vi "AutoApproach.vi"() -> ()   [LabVIEW 2014]
uses:
  <vilib>/userdefined/High Color/nirio_resource_hc.ctl
  <vilib>/Instr/_visa.llb/VISA Configure Serial Port (Instr).vi
  <vilib>/FPGAPlugInAG/PCIe-7851R/niLvFpga_Open_PCIe-7851R.vi
  <vilib>/rvi/interface/common/dynamic/niFpgaDynamicAddResources.vi
  <vilib>/Utility/error.llb/Error Cluster From Error Code.vi
  <vilib>/rvi/errors/niLvFpgaAdjustHostInterfaceError.vi
  <vilib>/FPGAPlugInAG/Dynamic/niLvFpga_Close_Dynamic.vi
  <vilib>/rvi/interface/nirviOpenFPGA/nirviOpenFPGA.xnode
  FPGA Bitfiles/FastHoppingModel_FPGATarget_CurrRefFres_BupT8kKEpOg.lvbitx
  <vilib>/rvi/interface/nirviReadWriteControl/nirviReadWriteControl.xnode
  <vilib>/rvi/interface/nirviCloseFPGA/nirviCloseFPGA.xnode
  FPGA Bitfiles/FastHoppingModel_FPGATarget_SingleApproach_ZxUoy3UGE18.lvbitx
  NiFpgaLv.dll
  <vilib>/rvi/interface/Simulation/niFpgaSimulationCallBeginRW.vi
panel:
  in  "RoughZOffset um":dbl format="%#_13g"
  out "Approached?":bool
  out "ERROut?":string
  in  "stop":bool
  out "RealPosIndex":i16
  out "preCurrIndex":i16
  out "PIZPosIndex":i16
  out "CurrDia":i16(graph)
  out "PIZPosDia":i16(graph)
  in  "Decline %":sgl format="%#_13g"
  in  "AppRate us":i32
  in  "BaseTime us":i32
  in  "PIZ":T1
  out "RoughZPos":dbl
  out "ERRIn?":string
  in  "RoughXYZ":refnum<visa-resource-name>
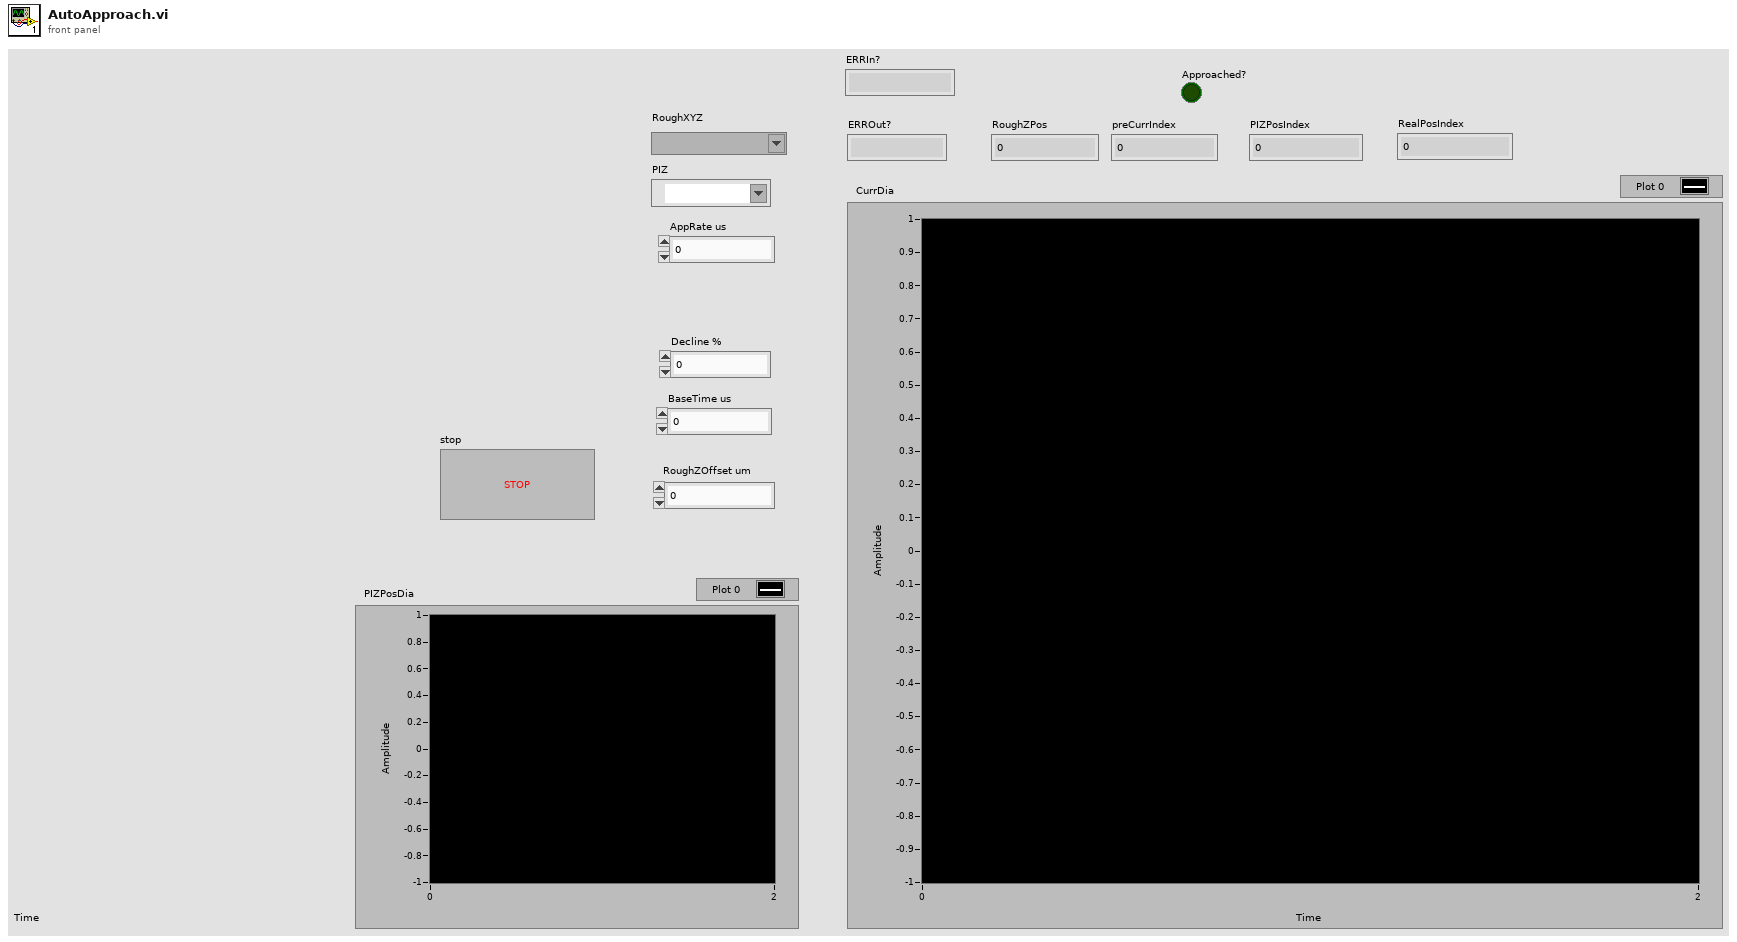
[diagram p1: front panel]
types:
  T1 = typedef "nirio_resource_hc.ctl" = tag
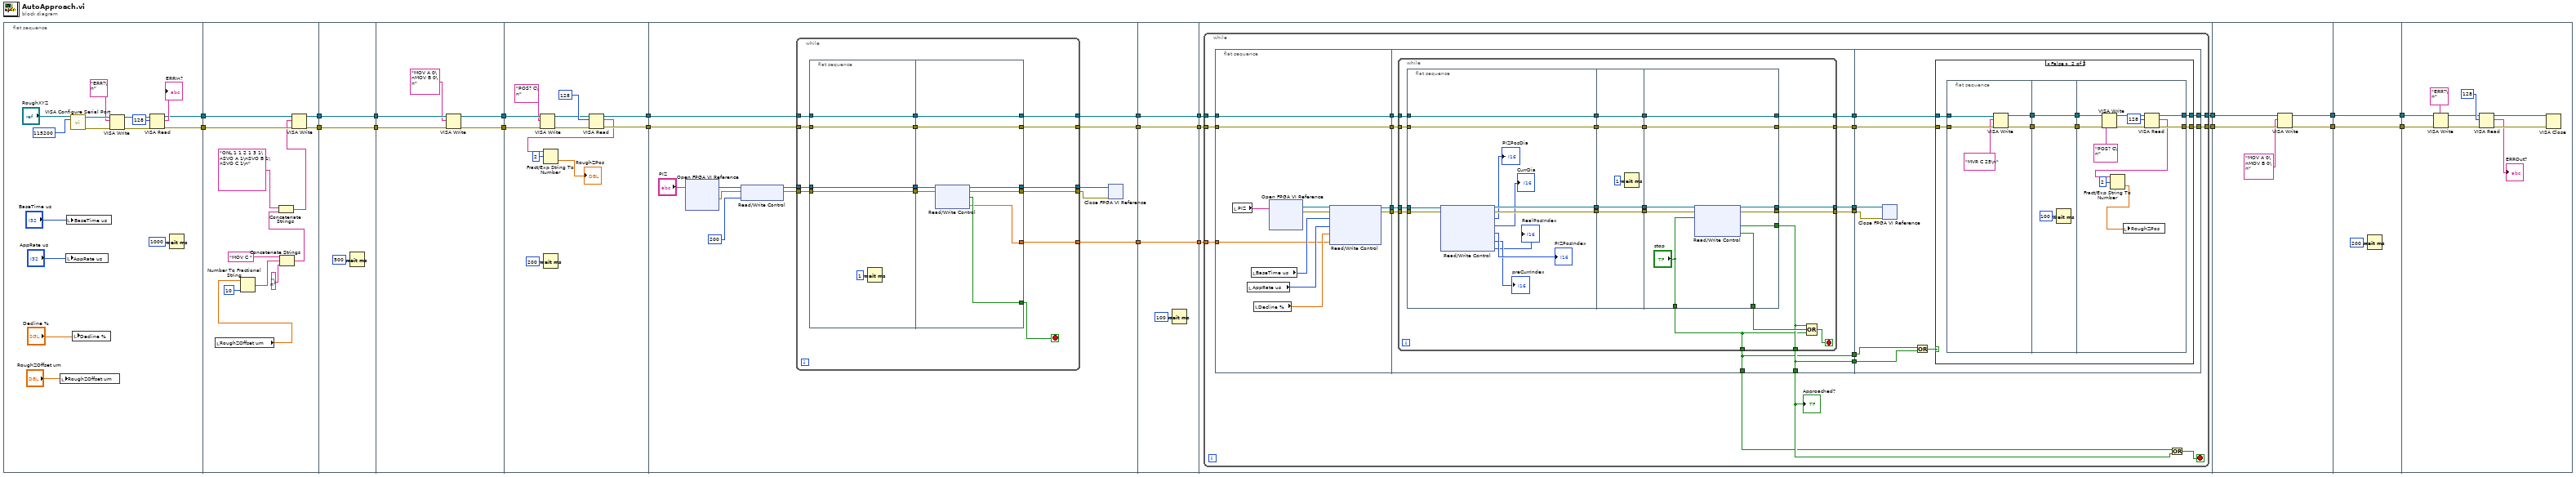
[diagram p0: block diagram]
diagram:
  n1 = flat-sequence {
    tunnel: [w29] -> w22
    tunnel: [w28] -> w21
    tunnel: w22 -> [w50]
    tunnel: w21 -> [w49]
    tunnel: [w48] -> w20
    tunnel: [w47] -> w19
    tunnel: w20 -> [w53]
    tunnel: w19 -> [w52]
    tunnel: [w53] -> w18
    tunnel: [w52] -> w17
    tunnel: w18 -> [w58]
    tunnel: w17 -> [w57]
    tunnel: [w56] -> w16
    tunnel: [w55] -> w15
    tunnel: w16 -> [w69]
    tunnel: w15 -> [w68]
    tunnel: [w63] -> w8
    tunnel: [w62] -> w7
    tunnel: w8 -> [w83]
    tunnel: [w78] -> w6
    tunnel: w7 -> [w82]
    tunnel: [w77] -> w4
    tunnel: [w72] -> w2
    tunnel: w6 -> [w114]
    tunnel: [w114] -> w5
    tunnel: w4 -> [w113]
    tunnel: [w113] -> w3
    tunnel: w2 -> [w112]
    tunnel: [w112] -> w1
    tunnel: w5 -> [w119]
    tunnel: w3 -> [w118]
    tunnel: [w117] -> w14
    tunnel: [w116] -> w13
    tunnel: w1 -> [w115]
    tunnel: w14 -> [w246]
    tunnel: w13 -> [w245]
    tunnel: [w243] -> w12
    tunnel: [w242] -> w11
    tunnel: w12 -> [w249]
    tunnel: w11 -> [w248]
    tunnel: [w249] -> w10
    tunnel: [w248] -> w9
    tunnel: w10 -> [w258]
    tunnel: w9 -> [w257]
    frame #0 {
      n2 = local write "RoughZOffset um"("RoughZOffset um") -> ()
      n3 = local write "AppRate us"("AppRate us") -> ()
      n4 = local write "BaseTime us"("BaseTime us") -> ()
      n5 = call-poly "VISA Configure Serial Port"("VISA resource name"="RoughXYZ", "baud rate (9600)"=u32 115200) -> ("VISA resource name out"=w36:refnum<visa-resource-name>, "error out"=w35:errorcluster)  [unwired: 12 in]
      n6 = local write "Decline %"("Decline %") -> ()
      n7 = VISA Write(VISA resource name=w36, write buffer="ERR?\n", error in (no error)=w35) -> (VISA resource name out=w33:refnum<visa-resource-name>, error out=w32:errorcluster)  [unwired: 1 out]
      n8 = VISA Read(VISA resource name=w33, byte count=u32 128, error in (no error)=w32) -> (VISA resource name out=w29:refnum<visa-resource-name>, read buffer=→"ERRIn?":string, error out=w28:errorcluster)  [unwired: 1 out]
      n9 = Wait (ms)(milliseconds to wait=u32 1000) -> ()  [unwired: 1 out]
    }
    frame #1 {
      n10 = local read "RoughZOffset um"() -> (w40:dbl)
      n11 = Number To Fractional String(number=w40, precision (6)=i16 10) -> (F-format string=w41:string)  [unwired: 2 in]
      n12 = Concatenate Strings("MOV C " ("string"), w41, "\n" ("string")) -> (w42:string)
      n13 = Concatenate Strings("ONL 1 1 2 1 3 1\nSVO A 1\nSVO B 1\nSVO C 1\n" ("write buffer"), w42) -> (w45:string)
      n14 = VISA Write(VISA resource name=w50, write buffer=w45, error in (no error)=w49) -> (VISA resource name out=w48:refnum<visa-resource-name>, error out=w47:errorcluster)  [unwired: 1 out]
    }
    frame #2 {
      n15 = Wait (ms)(milliseconds to wait=u32 500) -> ()  [unwired: 1 out]
    }
    frame #3 {
      n16 = VISA Write(VISA resource name=w58, write buffer="MOV A 0\nMOV B 0\n", error in (no error)=w57) -> (VISA resource name out=w56:refnum<visa-resource-name>, error out=w55:errorcluster)  [unwired: 1 out]
    }
    frame #4 {
      n17 = VISA Write(VISA resource name=w69, write buffer="POS? C\n", error in (no error)=w68) -> (VISA resource name out=w65:refnum<visa-resource-name>, error out=w64:errorcluster)  [unwired: 1 out]
      n18 = Wait (ms)(milliseconds to wait=u32 200) -> ()  [unwired: 1 out]
      n19 = VISA Read(VISA resource name=w65, byte count=u32 128, error in (no error)=w64) -> (VISA resource name out=w63:refnum<visa-resource-name>, read buffer=w61:string, error out=w62:errorcluster)  [unwired: 1 out]
      n20 = Fract/Exp String To Number(string=w61, offset=2) -> (number=→"RoughZPos":dbl)  [unwired: 2 in, 1 out]
    }
    frame #5 {
      n21 = xnode "Open FPGA VI Reference"("resource name"="PIZ") -> ("FPGA VI Reference Out"=w80:refnum<k20>, "error out"=w79:errorcluster)  [unwired: 1 in]
      n22 = xnode "Read/Write Control"("FPGA VI Reference In"=w80, "error in"=w79, "SampleNum"=200) -> ("FPGA VI Reference Out"=w76:refnum<k20>, "error out"=w75:errorcluster)
      n23 = while {
        tunnel: w83 -> [w96]
        tunnel: w82 -> [w93]
        tunnel: [w95] -> w78
        tunnel: [w92] -> w77
        tunnel: w76 -> [w91]
        tunnel: w75 -> [w90]
        tunnel: [w87] -> w74
        tunnel: [w86] -> w73
        tunnel: [w84] -> w72
        stop <- w85 stop-if-true
        n24 = flat-sequence {
          tunnel: [w102] -> w97
          tunnel: w96 -> [w102]
          tunnel: [w101] -> w94
          tunnel: w93 -> [w101]
          tunnel: w91 -> [w99]
          tunnel: w90 -> [w98]
          tunnel: [w99] -> w89
          tunnel: [w98] -> w88
          tunnel: w97 -> [w110]
          tunnel: [w110] -> w95
          tunnel: w94 -> [w109]
          tunnel: [w109] -> w92
          tunnel: w89 -> [w108]
          tunnel: w88 -> [w107]
          tunnel: [w106] -> w87
          tunnel: [w105] -> w86
          tunnel: [w104] -> w85
          tunnel: [w103] -> w84
          frame #0 {
            n25 = Wait (ms)(milliseconds to wait=u32 1) -> ()  [unwired: 1 out]
          }
          frame #1 {
            n26 = xnode "Read/Write Control"("FPGA VI Reference In"=w108, "error in"=w107) -> ("FPGA VI Reference Out"=w106:refnum<k20>, "error out"=w105:errorcluster, "Finished?"=w104:bool, "Ref"=w103:sgl)
          }
        }
      }
      n27 = xnode "Close FPGA VI Reference"("FPGA VI Reference In"=w74, "error in"=w73) -> ()  [unwired: 1 out]
    }
    frame #6 {
      n28 = Wait (ms)(milliseconds to wait=u32 100) -> ()  [unwired: 1 out]
    }
    frame #7 {
      n29 = while {
        tunnel: w119 -> [w135]
        tunnel: w118 -> [w134]
        tunnel: [w128] -> w117
        tunnel: [w127] -> w116
        tunnel: w115 -> [w120]
        stop <- w126 stop-if-true
        n30 = flat-sequence {
          tunnel: [w143] -> w137
          tunnel: [w142] -> w136
          tunnel: w135 -> [w141]
          tunnel: w134 -> [w140]
          tunnel: [w141] -> w133
          tunnel: [w140] -> w132
          tunnel: w120 -> [w138]
          tunnel: w137 -> [w158]
          tunnel: w136 -> [w157]
          tunnel: w133 -> [w156]
          tunnel: w132 -> [w155]
          tunnel: [w154] -> w131
          tunnel: [w153] -> w130
          tunnel: [w152] -> w125
          tunnel: [w152] -> w129
          tunnel: [w151] -> w124
          tunnel: [w151] -> w123
          tunnel: [w150] -> w122
          tunnel: [w149] -> w121
          tunnel: w131 -> [w212]
          tunnel: w130 -> [w211]
          tunnel: w129 -> [w204]
          tunnel: [w210] -> w128
          tunnel: [w209] -> w127
          tunnel: w123 -> [w205]
          tunnel: w122 -> [w208]
          tunnel: w121 -> [w207]
          frame #0 {
            n31 = local read "PIZ"() -> (w139:T1)
            n32 = local read "AppRate us"() -> (w145:i32)
            n33 = local read "BaseTime us"() -> (w146:i32)
            n34 = local read "Decline %"() -> (w144:sgl)
            n35 = xnode "Open FPGA VI Reference"("resource name"=w139) -> ("FPGA VI Reference Out"=w148:refnum<k20>, "error out"=w147:errorcluster)  [unwired: 1 in]
            n36 = xnode "Read/Write Control"("FPGA VI Reference In"=w148, "error in"=w147, "BaseTime us"=w146, "AppRate us"=w145, "Percentage %"=w144, "BaseCurrentRef"=w138) -> ("FPGA VI Reference Out"=w143:refnum<k20>, "error out"=w142:errorcluster)
          }
          frame #1 {
            n37 = while {
              tunnel: w158 -> [w178]
              tunnel: w157 -> [w177]
              tunnel: w156 -> [w174]
              tunnel: w155 -> [w173]
              tunnel: [w168] -> w154
              tunnel: [w167] -> w153
              tunnel: [w162] -> w152
              tunnel: [w161] -> w151
              tunnel: [w160] -> w150
              tunnel: [w159] -> w149
              stop <- w164 stop-if-true
              n38 = flat-sequence {
                tunnel: w178 -> [w189]
                tunnel: w177 -> [w188]
                tunnel: [w187] -> w176
                tunnel: [w186] -> w175
                tunnel: w174 -> [w180]
                tunnel: w173 -> [w179]
                tunnel: [w180] -> w172
                tunnel: [w179] -> w171
                tunnel: w176 -> [w191]
                tunnel: w175 -> [w190]
                tunnel: w172 -> [w193]
                tunnel: w171 -> [w192]
                tunnel: [w193] -> w170
                tunnel: [w192] -> w169
                tunnel: [w191] -> w166
                tunnel: [w190] -> w165
                tunnel: [w203] -> w168
                tunnel: w170 -> [w203]
                tunnel: [w202] -> w167
                tunnel: w169 -> [w202]
                tunnel: w166 -> [w201]
                tunnel: w165 -> [w200]
                tunnel: ["stop"] -> w161
                tunnel: [w198] -> w162
                tunnel: [w197] -> w163
                tunnel: [w196] -> w160
                tunnel: [w195] -> w159
                frame #0 {
                  n39 = xnode "Read/Write Control"("FPGA VI Reference In"=w189, "error in"=w188) -> ("FPGA VI Reference Out"=w187:refnum<k20>, "error out"=w186:errorcluster, "PIZPosIndexDia"=→"PIZPosDia":i16, "PreCurrIndexDia"=→"CurrDia":i16, "PIZPosIndex"=→"PIZPosIndex":i16, "preCurrIndex"=→"preCurrIndex":i16, "RealPosIndex"=→"RealPosIndex":i16)
                }
                frame #1 {
                  n40 = Wait (ms)(milliseconds to wait=u32 1) -> ()  [unwired: 1 out]
                }
                frame #2 {
                  n41 = xnode "Read/Write Control"("FPGA VI Reference In"=w201, "error in"=w200, "stop"="stop") -> ("FPGA VI Reference Out"=w196:refnum<k20>, "error out"=w195:errorcluster, "Approached?"=w198:bool, "Result"=w197:bool)
                }
              }
              n42 = Compound Arithmetic op=OR(w162, w163, w161) -> (w164:bool)
            }
          }
          frame #2 {
            n43 = xnode "Close FPGA VI Reference"("FPGA VI Reference In"=w208, "error in"=w207) -> ()  [unwired: 1 out]
            n44 = Or(x=w205, y=w204) -> (x .or. y?=w206:bool)
            n45 = case shown="False" w206 {
              tunnel: w212 -> [w214 w222]
              tunnel: w211 -> [w213 w221]
              tunnel: [w214 w216] -> w210
              tunnel: [w213 w215] -> w209
              frame True {
              }
              frame False {
                n46 = flat-sequence {
                  tunnel: w222 -> [w227]
                  tunnel: w221 -> [w226]
                  tunnel: [w224] -> w220
                  tunnel: [w223] -> w219
                  tunnel: w220 -> [w230]
                  tunnel: w219 -> [w229]
                  tunnel: [w230] -> w218
                  tunnel: [w229] -> w217
                  tunnel: w218 -> [w241]
                  tunnel: w217 -> [w240]
                  tunnel: [w236] -> w216
                  tunnel: [w235] -> w215
                  frame #0 {
                    n47 = VISA Write(VISA resource name=w227, write buffer="MVR C 25\n", error in (no error)=w226) -> (VISA resource name out=w224:refnum<visa-resource-name>, error out=w223:errorcluster)  [unwired: 1 out]
                  }
                  frame #1 {
                    n48 = Wait (ms)(milliseconds to wait=u32 100) -> ()  [unwired: 1 out]
                  }
                  frame #2 {
                    n49 = VISA Write(VISA resource name=w241, write buffer="POS? C\n", error in (no error)=w240) -> (VISA resource name out=w238:refnum<visa-resource-name>, error out=w237:errorcluster)  [unwired: 1 out]
                    n50 = VISA Read(VISA resource name=w238, byte count=u32 128, error in (no error)=w237) -> (VISA resource name out=w236:refnum<visa-resource-name>, read buffer=w233:string, error out=w235:errorcluster)  [unwired: 1 out]
                    n51 = Fract/Exp String To Number(string=w233, offset=2) -> (number=w231:dbl)  [unwired: 2 in, 1 out]
                    n52 = local write "RoughZPos"(w231) -> ()
                  }
                }
              }
            }
          }
        }
        n53 = Or(x=w124, y=w125) -> (x .or. y?=w126:bool)
        "Approached?" <- w125
      }
    }
    frame #8 {
      n54 = VISA Write(VISA resource name=w246, write buffer="MOV A 0\nMOV B 0\n", error in (no error)=w245) -> (VISA resource name out=w243:refnum<visa-resource-name>, error out=w242:errorcluster)  [unwired: 1 out]
    }
    frame #9 {
      n55 = Wait (ms)(milliseconds to wait=u32 200) -> ()  [unwired: 1 out]
    }
    frame #10 {
      n56 = VISA Write(VISA resource name=w258, write buffer="ERR?\n", error in (no error)=w257) -> (VISA resource name out=w254:refnum<visa-resource-name>, error out=w253:errorcluster)  [unwired: 1 out]
      n57 = VISA Read(VISA resource name=w254, byte count=u32 128, error in (no error)=w253) -> (VISA resource name out=w252:refnum<visa-resource-name>, read buffer=→"ERROut?":string, error out=w251:errorcluster)  [unwired: 1 out]
      n58 = VISA Close(VISA resource name=w252, error in (no error)=w251) -> ()  [unwired: 1 out]
    }
  }
